vi "DAE Radau 5th Order (Formula).vi"(7 "DAE F(X,X',t)":T2, 8 "error in (no error)":errorcluster, 9 "simulation parameters":T1={"initial time"=0.0, "final time"=10.0, "Absolute Tolerance"=[0.001], "Relative Tolerance"=[0.001], "minimum time step"=1e-08, "maximum time step"=1.0, "initial time step"=0.01} {"initial time step" min=0.0; "maximum time step" min=0.0; "minimum time step" min=0.0}, 10 "Initial Derivatives":dbl[](array[numeric]), 11 "Initial Values":dbl[](array[numeric])) -> (0 "error out":errorcluster, 1 "X Derivatives":dbl[][](array[numeric]), 2 "X Values":dbl[][](array[numeric]), 3 "Times":dbl[](array[numeric]))   [LabVIEW 2017, in "NI_DAE.lvlib"]
doc: "Solves differential algebraic equations (DAEs) with initial conditions by using the Radau IIA method. You must manually select the polymorphic instance to use."
uses:
  <vilib>/gmath/NI_DAE.lvlib
  <vilib>/gmath/dae.llb/Radau5_Parameters.ctl
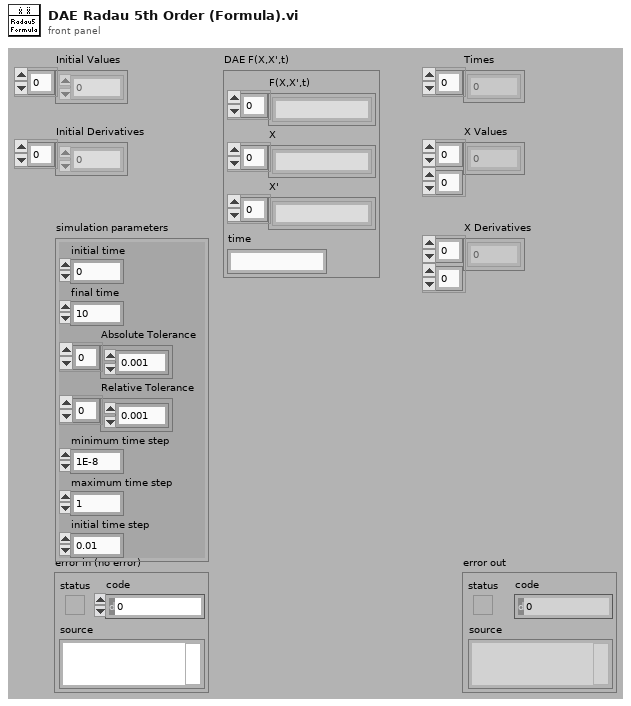
[diagram p1: front panel]
types:
  T1 = typedef "NI_DAE.lvlib/Radau5_Parameters.ctl" = cluster{"initial time":dbl, "final time":dbl, "Absolute Tolerance":dbl[], "Relative Tolerance":dbl[], "minimum time step":dbl, "maximum time step":dbl, "initial time step":dbl}
  T2 = cluster{"F(X,X',t)":string[], "X":string[], "X'":string[], "time":string}
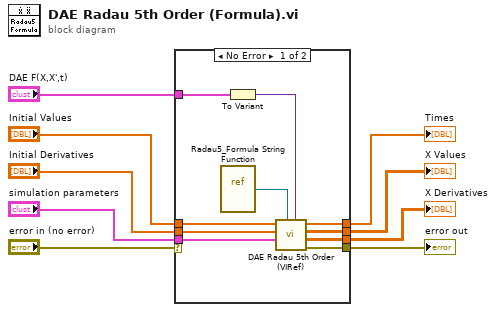
[diagram p0: block diagram]
diagram:
  n1 = case shown="No Error" "error in (no error)" {
    selector: "error in (no error)" -> [_ w20]
    tunnel: [w16 w20] -> w9
    tunnel: [w13 _] -> w8
    tunnel: [w14 _] -> w7
    tunnel: [w15 _] -> w6
    tunnel: "Initial Derivatives" -> [w18 _]
    tunnel: "Initial Values" -> [w19 _]
    tunnel: "simulation parameters" -> [w17 _]
    tunnel: "DAE F(X,X',t)" -> [w12 _]
    frame No Error {
      n2 = vi-ref <vilib>:"Radau5_Formula String Function.vi"() -> ("vi reference"=w10:refnum<vi>)
      n3 = To Variant(anything=w12) -> (Variant=w11:variant)
      n4 = call <vilib>:"DAE Radau 5th Order (VIRef).vi"("data"=w11, "DAE F(X,X',t)"=w10, "simulation parameters"=w17, "Initial Derivatives"=w18, "Initial Values"=w19) -> ("error out"=w16:errorcluster, "X Derivatives"=w15:dbl[][], "X Values"=w14:dbl[][], "Times"=w13:dbl[])  [unwired: 3 in]
    }
    frame Error {
    }
  }
  "Times" <- w8
  "X Values" <- w7
  "X Derivatives" <- w6
  "error out" <- w9
